vi "Test_020620t.vi"() -> ()   [LabVIEW 2020]
uses:
  d7c415e8-899e-4f39-80d6-ad140b58e363.vi
panel:
  out "size(s)":i32
  out "x/y":dbl
  out "XY Graph":cluster{"X":dbl, "Y":dbl}[](graph)
  in  "stop":bool
  in  "samples per second":dbl=1000.0
  in  "cycles":dbl=2.0
  in  "sampling":i32=1000
  out "Waveform Chart":dbl(graph)
  in  "offset (deg)":dbl format="%0.2p"
  in  "frequency":dbl=10.0 format="%0.2p"
  in  "amplitude":dbl=1.0 format="%0.2p"
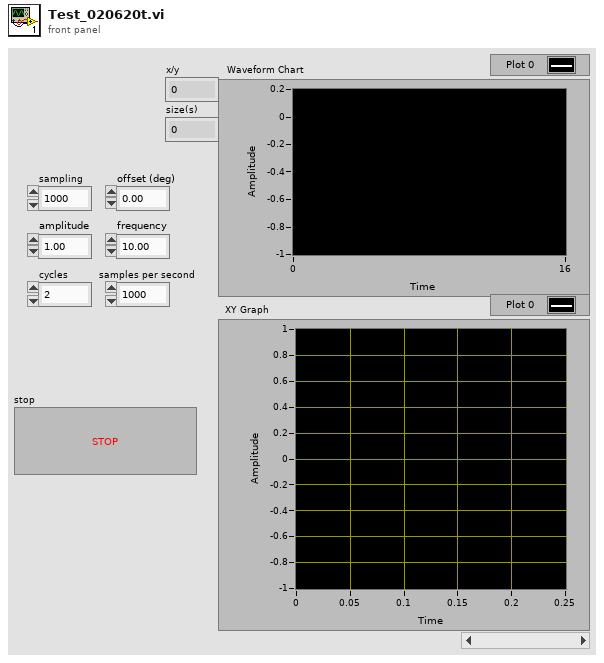
[diagram p1: front panel]
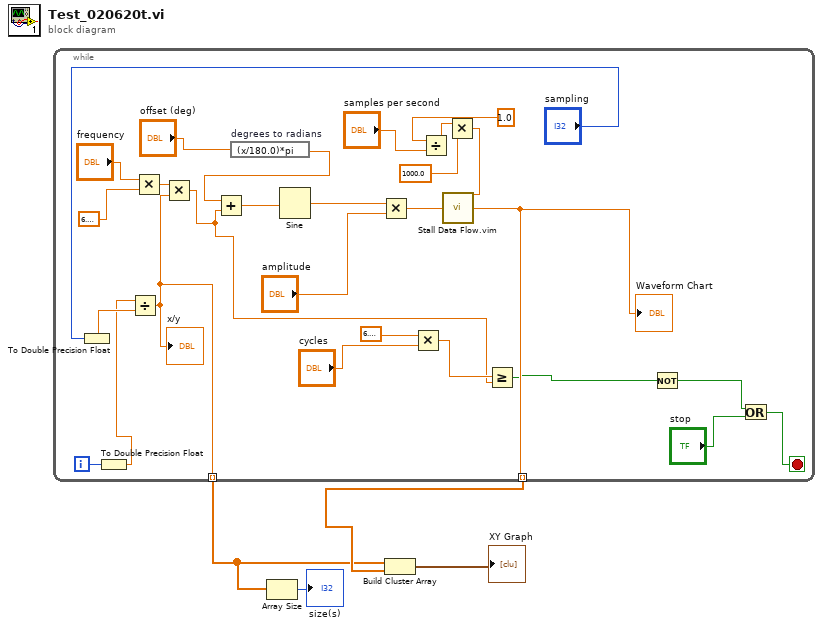
[diagram p0: block diagram]
diagram:
  n1 = while {
    tunnel: [w26] -> w3 mode=indexing
    tunnel: [w5] -> w2 mode=indexing
    i -> [w30]
    stop <- w15 stop-if-true
    n2 = To Double Precision Float(number="sampling") -> (double precision float=w28:dbl)
    n3 = To Double Precision Float(number=w30) -> (double precision float=w14:dbl)
    n4 = Divide(x=w14, y=w28) -> (x/y=w5:dbl)
    "x/y" <- w5
    n5 = Multiply(x="frequency", y=6.283185307179586) -> (x*y=w9:dbl)
    n6 = Multiply(x=w9, y=w5) -> (x*y=w8:dbl)
    n7 = expression code="(x/180.0)*pi" "degrees to radians"("offset (deg)") -> (w10:dbl)
    n8 = Add(x=w10, y=w8) -> (x+y=w29:dbl)
    n9 = Sine(x=w29) -> (sin(x)=w31:dbl)
    n10 = Multiply(x=w31, y="amplitude") -> (x*y=w27:dbl)
    n11 = Multiply(x=6.283185307179586, y="cycles") -> (x*y=w19:dbl)
    n12 = Divide(x=1.0, y="samples per second") -> (x/y=w23:dbl)
    n13 = Multiply(x=w23, y=1000.0) -> (x*y=w21:dbl)
    n14 = call "Stall Data Flow.vim"("value in"=w27, "milliseconds to wait"=w21) -> ("value out"=w26:dbl)  [unwired: 1 out]
    "Waveform Chart" <- w26
    n15 = Greater Or Equal?(x=w19, y=w8) -> (x >= y?=w18:bool)
    n16 = Not(x=w18) -> (.not. x?=w16:bool)
    n17 = Or(x=w16, y="stop") -> (x .or. y?=w15:bool)
  }
  n18 = Array Size(array=w2) -> (size(s)=→"size(s)":i32)
  n19 = Build Cluster Array(w2, w3) -> (→"XY Graph":cluster{dbl, "value out":dbl}[])
